vi "Map Events.vi"(8 "Error In":errorcluster) -> (0 "error out":errorcluster)   [LabVIEW 2014]
uses:
  Reference/SubVI/GMap DLL Refernce.vi
  C:/Robotic Systems/Products/AgFalcon/Software/Ground Station/Data/Mapping DLL/GMap.NET.WindowsForms.dll
  Data/Mapping DLL/GMap.NET.WindowsForms.dll
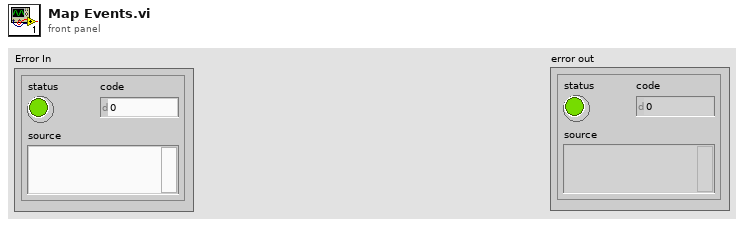
[diagram p1: front panel]
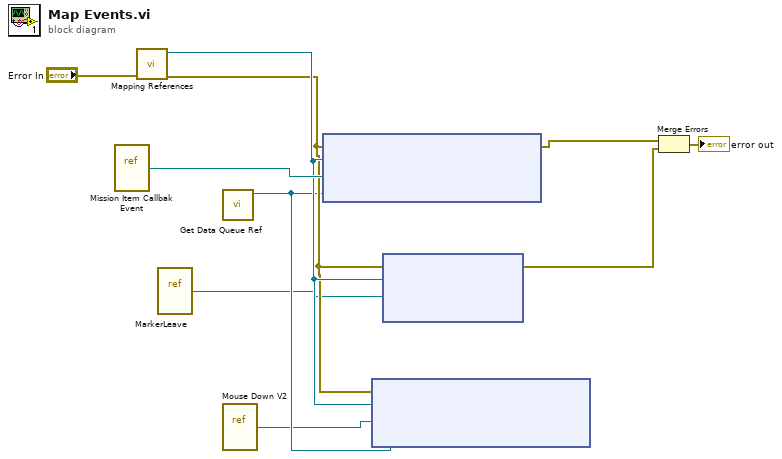
[diagram p0: block diagram]
diagram:
  n1 = vi-ref "Mission Item Callbak Event.vi"() -> ("vi reference"=w8:refnum<vi>)
  n2 = call-poly "Mapping References.vi"("Error In"="Error In") -> ("Error Out"=w4:errorcluster, "GMap DLL Reference"=w5:refnum<k24>)  [unwired: 9 in]
  n3 = vi-ref "MarkerLeave.vi"() -> ("vi reference"=w1:refnum<vi>)
  n4 = call "Get Data Queue Ref.vi"() -> ("Ground Station Operations Queue Ref"=w3:refnum<queue>)  [unwired: 10 in, 1 out]
  n5 = vi-ref "Mouse Down V2.vi"() -> ("vi reference"=w2:refnum<vi>)
  n6 = node(w4, w5, w8, w3) -> (w7:errorcluster)  [unwired: 1 in, 1 out]
  n7 = node(w4, w5, w2, w3) -> ()  [unwired: 1 in, 2 out]
  n8 = node(w4, w5, w1) -> (w6:errorcluster)  [unwired: 2 in, 1 out]
  n9 = Merge Errors(w7, w6) -> (→"error out":errorcluster)
